vi "get_config_cluster.vi"(8 "error in (no error)":errorcluster, 11 "FPGAWrapperRK120511Fiber_Spiral in":refnum<class "FPGAWrapperRK110512Fiber_Spiral.lvclass">) -> (0 "error out":errorcluster, 2 "config cluster (variant)":variant, 3 "FPGAWrapperRK120511Fiber_Spiral out":refnum<class "FPGAWrapperRK110512Fiber_Spiral.lvclass">)   [LabVIEW 2010, in "FPGAWrapperRK110512Fiber_Spiral.lvclass"]
uses:
  FPGAWrapperRK110512Fiber_Spiral.lvclass
  FPGAWrapperRK110512Fiber_Spiral.lvclass/FPGAWrapperRK110512Fiber_Spiral.ctl
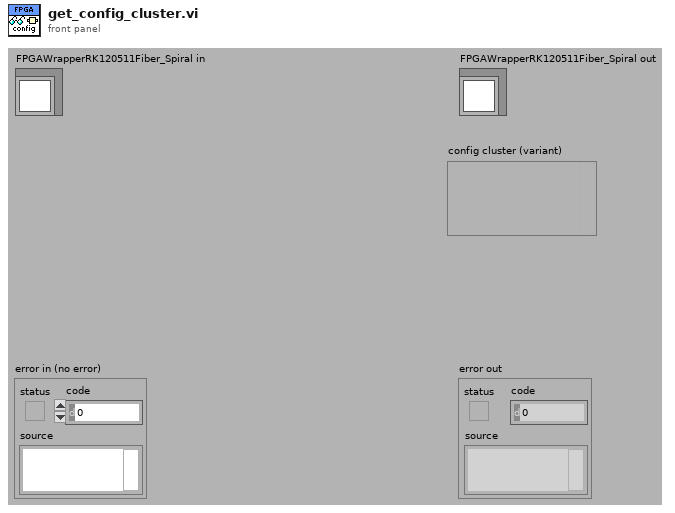
[diagram p1: front panel]
types:
  T1 = typedef "FPGAWrapperRK110512Fiber_Spiral.lvclass/config_data_cluster.ctl" = cluster{"Hifo box version":i16, "ADC clock phase":u8, "Enable ADC clock":bool, "FPGA Clock":u32}
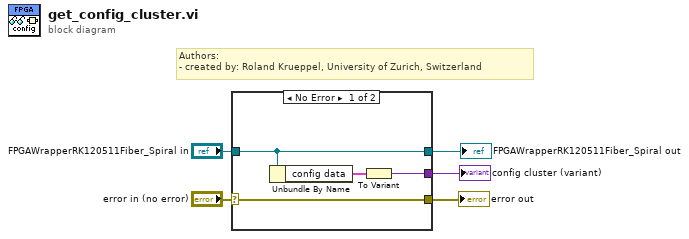
[diagram p0: block diagram]
diagram:
  # "Authors: \n- created by: Roland Krueppel, University of Zurich, Switzerland"
  n1 = case shown="No Error" "error in (no error)" {
    selector: "error in (no error)" -> [w6 w11]
    tunnel: "FPGAWrapperRK120511Fiber_Spiral in" -> [w8 w10]
    tunnel: [w8 w10] -> w3
    tunnel: [w6 w11] -> w2
    tunnel: [w7 _] -> w1
    frame No Error {
      n2 = Unbundle By Name(w8) -> ("config data"=w9:T1)
      n3 = To Variant(anything=w9) -> (Variant=w7:variant)
    }
    frame Error {
    }
  }
  "error out" <- w2
  "FPGAWrapperRK120511Fiber_Spiral out" <- w3
  "config cluster (variant)" <- w1
